vi "MTS_LaserController.vi"() -> ()   [LabVIEW 2011]
panel:
  out "Activity":bool
  in  "Act Red 2":bool=TRUE
  in  "Act Red 1":bool=TRUE
  in  "Act Blue 2":bool=TRUE
  in  "Act Blue 1":bool=TRUE
  in  "Blue Power":bool
  in  "Red Power":bool
  in  "Red Laser 2":dbl(slide) min=0.0 max=100.0 step=0.1 scale=0.0..100.0 scale format="%.1f %%"
  in  "Red Laser 1":dbl(slide) min=0.0 max=100.0 step=0.1 scale=0.0..100.0 scale format="%.1f %%"
  in  "Green Laser 2":dbl(slide) min=0.0 max=100.0 step=0.1 scale=0.0..100.0 scale format="%.1f %%"
  in  "Green Laser 1":dbl(slide) min=0.0 max=100.0 step=0.1 scale=0.0..100.0 scale format="%.1f %%"
  in  "Blue Laser 2":dbl(slide) min=0.0 max=100.0 step=0.1 scale=0.0..100.0 scale format="%.1f %%"
  out "Detector3":bool
  out "Detector4":bool
  out "Init Error":u32
  out "Intensity (a.u.)":dbl
  out "Close Error Number":u32 format="%.0x"
  in  "Init/Deint Can":bool=TRUE
  out "Excitation":bool
  out "Detector1":bool
  out "Detector2":bool
  out "Intensity (a.u.)":dbl=1.0 format="%.02f"
  in  "Blue Laser 1":dbl(slide) min=0.0 max=100.0 step=0.1 scale=0.0..100.0 scale format="%.1f %%"
  out "Laser 5 pos.":u16
  out "Laser 6 pos.":u16
  out "Laser 7 pos.":u16
  out "Laser 8 pos.":u16
  out "Laser 4 pos.":u16
  out "Laser 3 pos.":u16
  out "Laser 2 pos.":u16
  out "Laser 1 pos.":u16
  in  "stop":bool
  # "Laser Power Adjustment"
  # "BLUE"
  # "GREEN"
  # "RED"
  # "Positions"
  # "(470 nm)"
  # "(532 nm)"
  # "(640 nm)"
  # "Shutter"
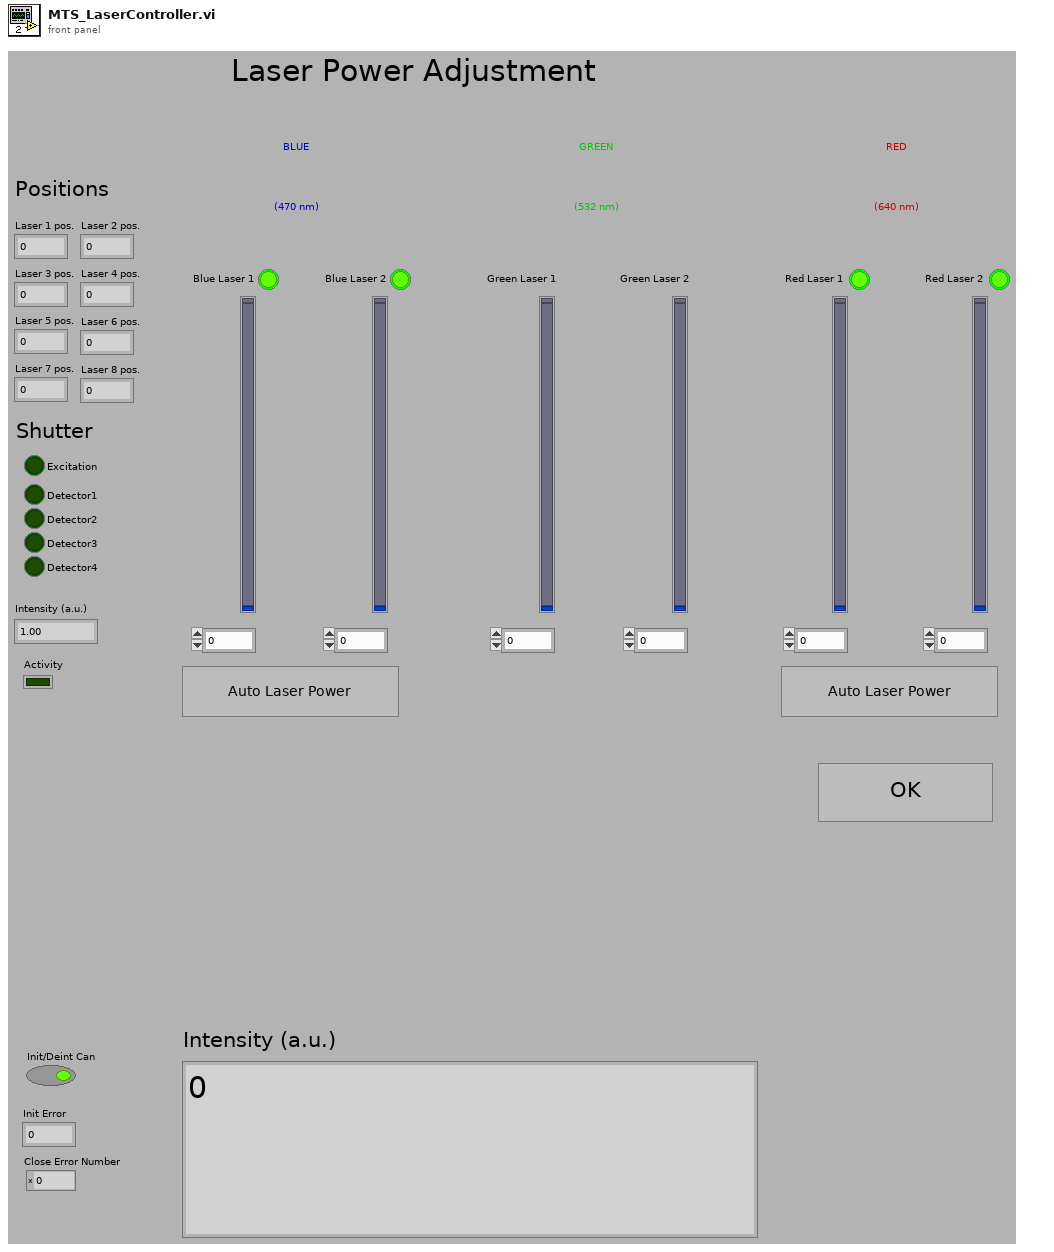
[diagram p1: front panel]
types:
  T1 = enum16{"CAN_Baud_1M", "CAN_BAUD_500K", "CAN_BAUD_250K", "CAN_BAUD_125K", "CAN_BAUD_100K", "CAN_BAUD_50K", "CAN_BAUD_20K", "CAN_BAUD_10K", "CAN_BAUD_5K", "User"}
  T2 = cluster{"ID":u32, "MSG type":enum8{"STD, NO RTR", "STD,RTR", "XTD, NO RTR", "XTD, RTR"}, "LEN":u8, "DATA":u8[]}
  T3 = enum8{"STD, NO RTR", "STD,RTR", "XTD, NO RTR", "XTD, RTR"}
  T4 = cluster{"x":u32, "MSG type":enum8{"STD, NO RTR", "STD,RTR", "XTD, NO RTR", "XTD, RTR"}, "LEN 3":u8, "Array":u8[]}
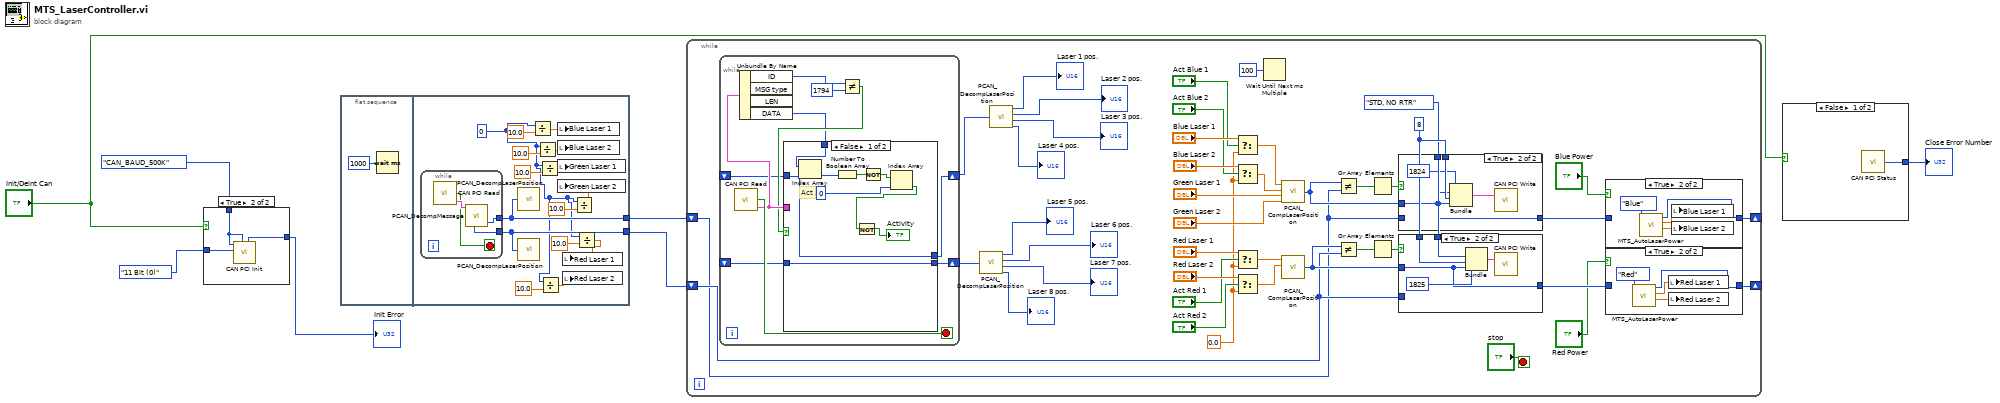
[diagram p0: block diagram]
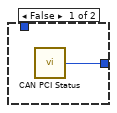
[diagram p2: hidden frame]
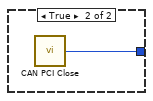
[diagram p3: hidden frame]
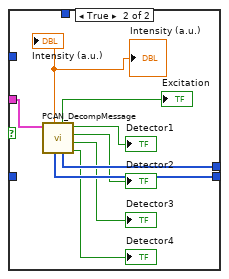
[diagram p8: hidden frame]
diagram:
  n1 = case shown="True" "Init/Deint Can" {
    tunnel: enum16{"11 Bit (0)", "29/11 Bit (1)"}."11 Bit (0)" ("CAN Msg Type") -> [_ w11]
    tunnel: T1."CAN_BAUD_500K" ("BTR0BTR1") -> [_ w10]
    tunnel: [w8 w9] -> w1
    frame False {
      n2 = call "CAN PCI Status.vi"() -> ("Error Number"=w8:u32)  [unwired: 1 in]
    }
    frame True {
      n3 = call "CAN PCI Init.vi"("BTR0BTR1(User)"=w10, "CAN Msg Type"=w11, "BTR0BTR1"=w10) -> ("Error Number"=w9:u32)  [unwired: 6 in, 2 out]
    }
  }
  "Init Error" <- w1
  n4 = flat-sequence {
    tunnel: [w26] -> w6
    tunnel: [w27] -> w5
    frame #0 {
      n5 = Wait (ms)(milliseconds to wait=u32 1000) -> ()  [unwired: 1 out]
    }
    frame #1 {
      w13 = u16 0 ("Laser 1 pos.")
      n6 = while {
        tunnel: [w29] -> w26
        tunnel: [w28] -> w27
        stop <- w30 stop-if-true
        n7 = call "CAN PCI Read.vi"() -> ("RcvQueueEmpty"=w30:bool, "CAN_Message out"=w31:T2)  [unwired: 1 in, 1 out]
        n8 = call "PCAN_DecompMessage.vi"("CAN_Message out"=w31) -> ("Laser 1-4"=w29:u8[], "Laser 5-8"=w28:u8[])  [unwired: 3 in, 6 out]
      }
      n9 = call "PCAN_DecompLaserPosition.vi"("DATA"=w26) -> ()  [unwired: 4 out]
      n10 = call "PCAN_DecompLaserPosition.vi"("DATA"=w27) -> ()  [unwired: 4 out]
      n11 = Divide(x=w13, y=10.0) -> (x/y=w24:dbl)
      n12 = Divide(x=w13, y=10.0) -> (x/y=w18:dbl)
      n13 = Divide(x=w13, y=10.0) -> (x/y=w19:dbl)
      n14 = Divide(x=w13, y=10.0) -> (x/y=w14:dbl)
      n15 = local write "Blue Laser 1"(w24) -> ()
      n16 = local write "Blue Laser 2"(w18) -> ()
      n17 = local write "Green Laser 1"(w19) -> ()
      n18 = local write "Red Laser 2"(w14) -> ()
      n19 = Divide(x=w13, y=10.0) -> (x/y=w20:dbl)
      n20 = local write "Green Laser 2"(w20) -> ()
      n21 = Divide(x=w13, y=10.0) -> (x/y=w15:dbl)
      n22 = local write "Red Laser 1"(w15) -> ()
    }
  }
  n23 = while {
    shift-right: [w50] -> _
    shift-left: w6 -> [w53]
    shift-right: [w49] -> _
    shift-left: w5 -> [w58]
    stop <- "stop" stop-if-true
    w32 = 0.0 ("f")
    w63 = T3."STD, NO RTR" ("MSG type")
    w72 = u8 8 ("LEN 3")
    n24 = while {
      shift-right: [w104] -> w61
      shift-left: _ -> [w99]
      shift-right: [w105] -> w62
      shift-left: _ -> [w98]
      stop <- w106 stop-if-true
      n25 = call "CAN PCI Read.vi"() -> ("RcvQueueEmpty"=w106:bool, "CAN_Message out"=w103:T2)  [unwired: 1 in, 1 out]
      n26 = Unbundle By Name(w103) -> ("ID"=w102:u32, "DATA"=w97:u8[])  [unwired: 2 out]
      n27 = Not Equal?(x=w102, y=u32 1794) -> (x != y?=w100:bool)
      n28 = case shown="False" w100 {
        tunnel: w103 -> [_ w124]
        tunnel: [w114 w123] -> w105
        tunnel: [w115 w122] -> w104
        tunnel: w99 -> [w115 _]
        tunnel: w98 -> [w114 _]
        tunnel: w97 -> [w109 _]
        frame False {
          # "Act"
          n29 = Index Array(array=w109) -> (element=w113:u8)  [unwired: 1 in]
          n30 = Number To Boolean Array(number=w113) -> (Boolean array=w112:bool[])
          n31 = Not(x=w112) -> (.not. x?=w111:bool[])
          n32 = Index Array(array=w111, index=0 ("y")) -> (element=w108:bool)
          n33 = Not(x=w108) -> (.not. x?=→"Activity":bool)
        }
        frame True {
          n34 = call "PCAN_DecompMessage.vi"("CAN_Message out"=w124) -> ("Detector4 Shutter Open?"=→"Detector4":bool, "Detector3 Shutter Open?"=→"Detector3":bool, "Detector2 Shutter Open?"=→"Detector2":bool, "Detector1 Shutter Open?"=→"Detector1":bool, "Laser 1-4"=w123:u8[], "Excitation Shutter Open?"=→"Excitation":bool, "Laser 5-8"=w122:u8[], "Intensity (a.u.)"=→"Intensity (a.u.)" →"Intensity (a.u.)":dbl)  [unwired: 3 in]
        }
      }
    }
    n35 = call "PCAN_DecompLaserPosition.vi"("DATA"=w61) -> ("Laser 1 pos."=→"Laser 5 pos.":u16, "Laser 2 pos."=→"Laser 6 pos.":u16, "Laser 3 pos."=→"Laser 7 pos.":u16, "Laser 4 pos."=→"Laser 8 pos.":u16)
    n36 = call "PCAN_DecompLaserPosition.vi"("DATA"=w62) -> ("Laser 1 pos."=→"Laser 1 pos.":u16, "Laser 2 pos."=→"Laser 2 pos.":u16, "Laser 3 pos."=→"Laser 3 pos.":u16, "Laser 4 pos."=→"Laser 4 pos.":u16)
    n37 = Select(t="Blue Laser 1", s="Act Blue 1", f=w32) -> (s? t:f=w38:dbl)
    n38 = Select(t="Blue Laser 2", s="Act Blue 2", f=w32) -> (s? t:f=w37:dbl)
    n39 = Select(t="Red Laser 1", s="Act Red 1", f=w32) -> (s? t:f=w40:dbl)
    n40 = Select(t="Red Laser 2", s="Act Red 2", f=w32) -> (s? t:f=w39:dbl)
    n41 = Wait Until Next ms Multiple(millisecond multiple=u32 100) -> ()  [unwired: 1 out]
    n42 = call "PCAN_CompLaserPosition.vi"("Laser 4"="Green Laser 2", "Laser 3"="Green Laser 1", "Laser 2"=w37, "Laser 1"=w38) -> ("Array"=w60:u8[])
    n43 = call "PCAN_CompLaserPosition.vi"("Laser 2"=w39, "Laser 1"=w40) -> ("Array"=w59:u8[])  [unwired: 2 in]
    n44 = Not Equal?(x=w60, y=w53) -> (x != y?=w57:bool[])
    n45 = Not Equal?(x=w59, y=w58) -> (x != y?=w55:bool[])
    n46 = Or Array Elements(Boolean array=w57) -> (logical OR=w56:bool)
    n47 = Or Array Elements(Boolean array=w55) -> (logical OR=w54:bool)
    n48 = case shown="True" w56 {
      tunnel: w72 -> [_ w95]
      tunnel: w63 -> [_ w94]
      tunnel: w60 -> [_ w92]
      tunnel: [w91 w92] -> w51
      tunnel: w53 -> [w91 _]
      frame False {
      }
      frame True {
        n49 = Bundle("x"=u32 1824, "MSG type"=w94, "LEN 3"=w95, "Array"=w92) -> (w96:T4)  [unwired: 1 in]
        n50 = call "CAN PCI Write.vi"("CAN_Message"=w96) -> ()  [unwired: 2 in, 1 out]
      }
    }
    n51 = case shown="True" w54 {
      tunnel: w72 -> [_ w88]
      tunnel: w63 -> [_ w87]
      tunnel: w59 -> [_ w86]
      tunnel: [w85 w86] -> w48
      tunnel: w58 -> [w85 _]
      frame False {
      }
      frame True {
        n52 = Bundle("x"=u32 1825, "MSG type"=w87, "LEN 3"=w88, "Array"=w86) -> (w89:T4)  [unwired: 1 in]
        n53 = call "CAN PCI Write.vi"("CAN_Message"=w89) -> ()  [unwired: 2 in, 1 out]
      }
    }
    n54 = case shown="True" "Blue Power" {
      tunnel: w51 -> [w80 _]
      tunnel: [w80 w83] -> w50
      frame False {
      }
      frame True {
        n55 = call "MTS_AutoLaserPower.vi"("Laser Color"=enum16{"Blue", "Green", "Red"}."Blue") -> ("Laser 2 Position"=w81:dbl, "Laser 1 Position"=w82:dbl, "New Positions"=w83:u8[])  [unwired: 7 in, 1 out]
        n56 = local write "Blue Laser 1"(w82) -> ()
        n57 = local write "Blue Laser 2"(w81) -> ()
      }
    }
    n58 = case shown="True" "Red Power" {
      tunnel: w48 -> [w75 _]
      tunnel: [w75 w78] -> w49
      frame False {
      }
      frame True {
        n59 = call "MTS_AutoLaserPower.vi"("Laser Color"=enum16{"Blue", "Green", "Red"}."Red") -> ("Laser 2 Position"=w76:dbl, "Laser 1 Position"=w77:dbl, "New Positions"=w78:u8[])  [unwired: 7 in, 1 out]
        n60 = local write "Red Laser 1"(w77) -> ()
        n61 = local write "Red Laser 2"(w76) -> ()
      }
    }
  }
  n62 = case shown="False" "Init/Deint Can" {
    tunnel: [w125 w126] -> w7
    frame False {
      n63 = call "CAN PCI Status.vi"() -> ("Error Number"=w125:u32)  [unwired: 1 in]
    }
    frame True {
      n64 = call "CAN PCI Close.vi"() -> ("Error Number"=w126:u32)  [unwired: 1 in]
    }
  }
  "Close Error Number" <- w7
